vi "Convergence Study (Trap).vi"() -> ()   [LabVIEW 2017]
panel:
  in  "Digitizing Parameters":T1={"Number of Samples"=1000, "Lower Limit"=0.0, "Upper Limit"=5.0}
  in  "Function Parameters":cluster{"Prefactor":dbl, "Power":dbl}={"Prefactor"=0.0, "Power"=2.0}
  out "XY Graph":cluster{i32[], dbl[]}(graph)
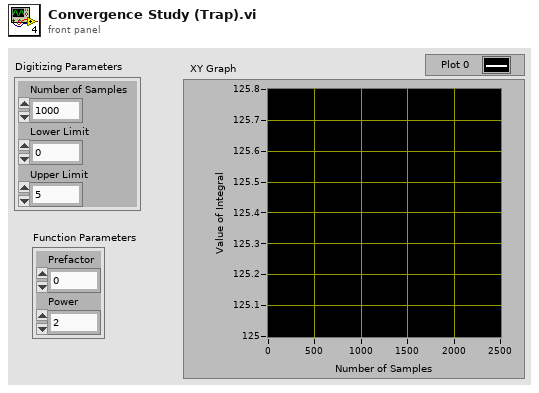
[diagram p1: front panel]
types:
  T1 = cluster{"Number of Samples":i32, "Lower Limit":dbl, "Upper Limit":dbl}
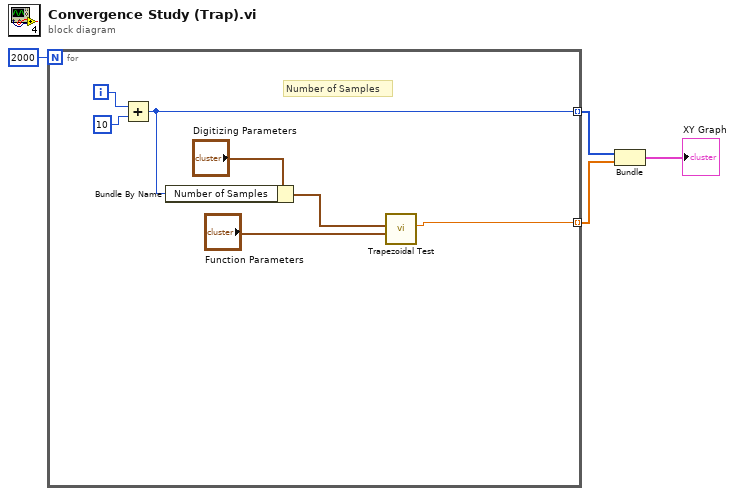
[diagram p0: block diagram]
diagram:
  n1 = for {
    N: 2000 -> [_]
    tunnel: [w6] -> w3 mode=indexing
    tunnel: [w8] -> w2 mode=indexing
    i -> [w10]
    # "Number of Samples"
    n2 = Add(x=w10, y=10) -> (x+y=w6:i32)
    n3 = Bundle By Name(cluster="Digitizing Parameters", "Number of Samples"=w6) -> (w5:T1)
    n4 = call "Trapezoidal Test.vi"("Function Parameters"="Function Parameters", "Digitizing Parameters"=w5) -> ("Value of Integral"=w8:dbl)  [unwired: 9 in]
  }
  n5 = Bundle(w3, w2) -> (→"XY Graph":cluster{i32[], dbl[]})  [unwired: 1 in]
